vi "get_volumes_listbox_items.vi"(11 "Volumes in":refnum<class "CLZ Comics.lvclass">) -> (2 "listbox items":string[][](array[string]), 3 "Volumes out":refnum<class "CLZ Comics.lvclass">)   [LabVIEW 2024, in "CLZ_to_ComicVine.lvlib" / "CLZ Comics.lvclass"]
uses:
  CLZ Comics.lvclass
  CLZ Comics.lvclass/CLZ Comics.ctl
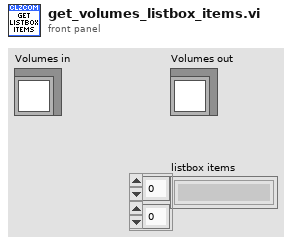
[diagram p1: front panel]
types:
  T1 = typedef "CLZ_to_ComicVine.lvlib/CLZ Comics.lvclass/volume--cluster.ctl" = cluster{"id":i32, "name":string, "issues":T2[], "matched":bool}
  T2 = typedef "CLZ_to_ComicVine.lvlib/CLZ Comics.lvclass/issue_number--cluster.ctl" = cluster{"numeric":dbl, "issue":string, "variant":string}
  T3 = cluster{"string out":string, "f":string, string, string}
  T4 = cluster{"string out":string, "f":string, string, string}[]
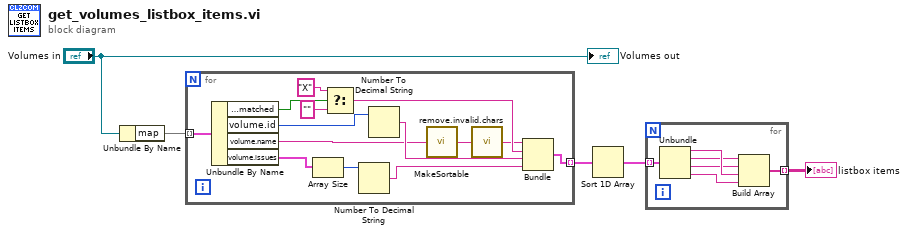
[diagram p0: block diagram]
diagram:
  n1 = Unbundle By Name("Volumes in") -> ("map"=w5:map{i32, T1})
  n2 = for {
    tunnel: w5 -> [w19] mode=indexing
    tunnel: [w9] -> w3 mode=indexing
    n3 = Unbundle By Name(w19) -> ("volume.matched"=w16:bool, "volume.id"=w15:i32, "volume.name"=w6:string, "volume.issues"=w14:T2[])
    n4 = Array Size(array=w14) -> (size(s)=w13:i32)
    n5 = Select(t="X", s=w16, f="") -> (s? t:f=w12:string)
    n6 = Number To Decimal String(number=w13) -> (decimal integer string=w10:string)  [unwired: 1 in]
    n7 = Number To Decimal String(number=w15) -> (decimal integer string=w11:string)  [unwired: 1 in]
    n8 = call "MakeSortable.vi"("string in"=w6) -> ("string out"=w8:string)
    n9 = call "remove.invalid.chars.vi"("string in"=w8) -> ("string out"=w7:string)
    n10 = Bundle("string out"=w7, "f"=w12, w11, w10) -> (w9:T3)  [unwired: 1 in]
  }
  n11 = Sort 1D Array(array=w3) -> (sorted array=w2:T4)
  n12 = for {
    tunnel: w2 -> [w25] mode=indexing
    tunnel: [w24] -> w1 mode=indexing
    n13 = Unbundle(w25) -> ("string out"=w23:string, "f"=w22:string, w21:string, w20:string)
    n14 = Build Array(w22, w21, w23, w20) -> (w24:string[])
  }
  "listbox items" <- w1
  "Volumes out" <- "Volumes in"
